vi "SpeakEngine.vi"(8 "error in (no error)":errorcluster, 9 "Text to speak":string="May the force be with you", 10 "EnumSpeak":T1) -> (0 "error out":errorcluster)   [LabVIEW 8.6]
uses:
  EnumSpeak.ctl
panel:
  in  "Voice":u16(ring) items=["Microsoft Sam"]
  in  "Audio Device":u16(ring) items=["SigmaTel Audio"]
  in  "Rate":i32(slide) scale=-10.0..10.0
  in  "Volume":i32(slide)=100 scale=0.0..100.0
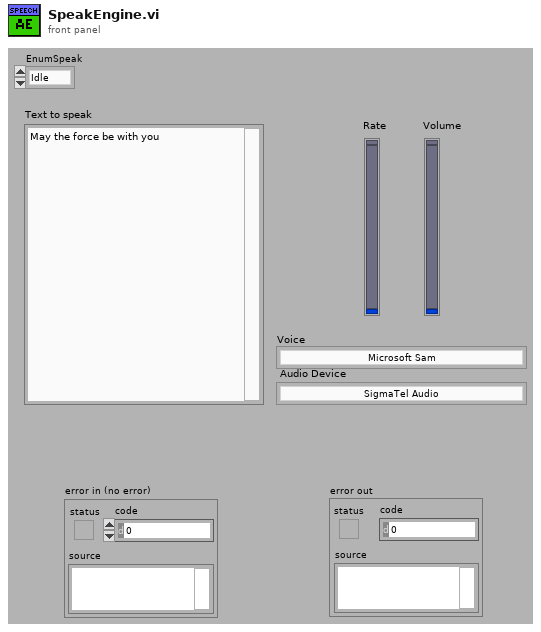
[diagram p1: front panel]
types:
  T1 = typedef "EnumSpeak.ctl" = enum16{"Idle", "Init", "Speak", "Close"}
  T2 = cluster{"SpeechLib.ISpeechVoice":refnum<k7>, "GetVoices":refnum<k7>, "GetAudioOutputs":refnum<k7>}
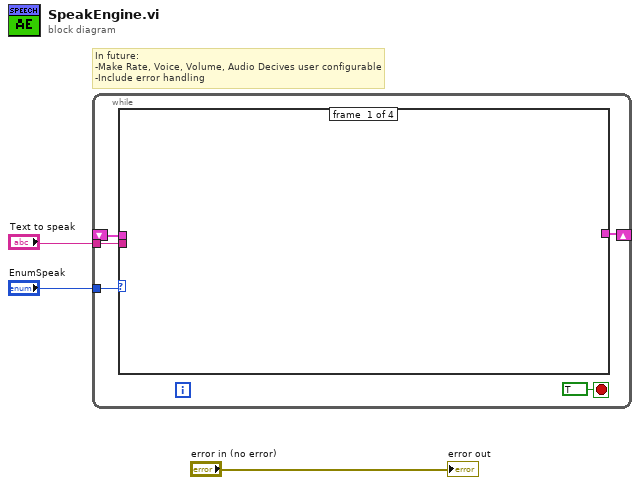
[diagram p0: block diagram]
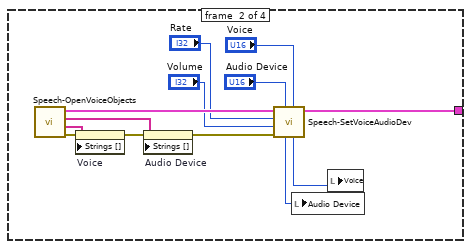
[diagram p2: hidden frame]
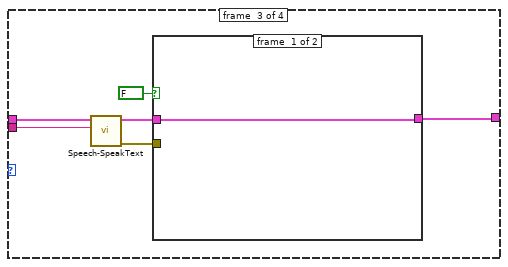
[diagram p3: hidden frame]
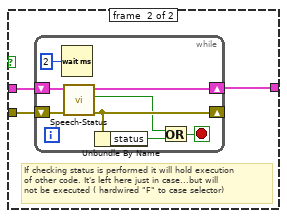
[diagram p4: hidden frame]
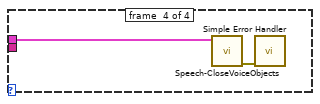
[diagram p5: hidden frame]
diagram:
  # "In future:\n-Make Rate, Voice, Volume, Audio Decives user configurable\n-Include error handling"
  n1 = while {
    tunnel: "EnumSpeak" -> [w7]
    shift-right: [w6] -> _
    shift-left: _ -> [w5]
    tunnel: "Text to speak" -> [w4]
    stop <- TRUE ("stop") stop-if-true
    n2 = case shown="\"Speak\"" w7 {
      tunnel: [_ w9 w24 _] -> w6
      tunnel: w5 -> [_ _ w25 w40]
      tunnel: w4 -> [_ _ w23 _]
      frame #0 {
      }
      frame #1 {
        n3 = call "Speech-OpenVoiceObjects.vi"() -> ("error out"=w19:errorcluster, "Voice Names"=w21:string[], "AudioDevices"=w20:string[], "speech_voice_refs"=w14:T2)  [unwired: 8 in]
        n4 = property on="Voice" class="Ring (strict)"(error in=w19, "Strings []"=w21) -> (error out=w18:errorcluster)  [unwired: 1 in, 1 out]
        n5 = property on="Audio Device" class="Ring (strict)"(error in=w18, "Strings []"=w20) -> (error out=w17:errorcluster)  [unwired: 1 in, 1 out]
        n6 = call "Speech-SetVoiceAudioDev.vi"("Voice"="Voice", "Audio Device"="Audio Device", "error in"=w17, "Volume"="Volume", "Rate"="Rate", "speech_voice_refs"=w14) -> ("speech_voice_refs (out)"=w9:T2, "Voice (out)"=w12:u16, "AudioDevice (out)"=w13:u16)  [unwired: 2 in, 1 out]
        n7 = local write "Audio Device"(w13) -> ()
        n8 = local write "Voice"(w12) -> ()
      }
      frame #2 {
        n9 = call "Speech-SpeakText.vi"("text to be spoken"=w23, "speech_voice_refs (in)"=w25) -> ("error out"=w26:errorcluster, "speech_voice_refs (out)"=w27:T2)  [unwired: 8 in]
        n10 = case shown="False" FALSE {
          tunnel: w27 -> [w28 w31]
          tunnel: w26 -> [_ w30]
          tunnel: [w28 w29] -> w24
          frame #0 {
          }
          frame #1 {
            # "If checking status is performed it will hold execution\nof other code. It's left here just in case...but will\nnot be executed ( hardwired \"F\" to case selector)"
            n11 = while {
              shift-right: [w34] -> _
              shift-left: w30 -> [w38]
              shift-right: [w35] -> w29
              shift-left: w31 -> [w39]
              stop <- w36 stop-if-true
              n12 = Wait (ms)(milliseconds to wait=u32 2) -> ()  [unwired: 1 out]
              n13 = call "Speech-Status.vi"("error in (no error)"=w38, "speech_voice_refs"=w39) -> ("error out"=w34:errorcluster, "Status (T: Done)"=w33:bool, "speech_voice_refs (out)"=w35:T2)  [unwired: 7 in]
              n14 = Unbundle By Name(w34) -> ("status"=w37:bool)
              n15 = Or(x=w33, y=w37) -> (x .or. y?=w36:bool)
            }
          }
        }
      }
      frame #3 {
        n16 = call "Speech-CloseVoiceObjects.vi"("speech object references"=w40) -> ("error out"=w41:errorcluster)  [unwired: 10 in]
        n17 = call <vilib>:"Simple Error Handler.vi"("error in (no error)"=w41) -> ()  [unwired: 4 in, 5 out]
      }
    }
  }
  "error out" <- "error in (no error)"
